vi "Read CAN Frame.vi"(8 "error in (no error)":errorcluster, 10 "Header Read":T3, 11 "BLF File In":refnum<class "Read Write BLF.lvclass">) -> (0 "error out":errorcluster, 1 "CAN Channel":u16, 2 "CAN Frame":T1 {"type" items=["CAN Data"=0, "CAN Remote"=1, "CAN Bus Error"=2, "CAN 2.0 Data"=8, "CAN FD Data"=16, "CAN FD+BRS Data"=24, "J1939 Data"=192, "Delay"=224, "Log Trigger"=225, "Start Trigger"=226]; "payload" format="%x"; "timestamp" format="%<%.7X\n%x>T"; "identifier" format="%x"}, 3 "BLF File Out":refnum<class "Read Write BLF.lvclass">)   [LabVIEW 2015, in "Read Write BLF.lvclass"]
doc: "This is the private function that will read a single <B>CAN Frame</B> given the header information of the next object position.\n\n-------------\nBrian Hoover (Hooovahh)"
uses:
  Read Write BLF.lvclass
  Controls/Cluster - mHeaderBase.ctl
  Controls/Enum - Read Object Types.ctl
  Controls/Cluster - CAN Frame.ctl
  Controls/Enum - CAN Data Type.ctl
  Read Write BLF.lvclass/Read Write BLF.ctl
  Controls/Cluster - CAN Message.ctl
  Controls/Cluster - mHeader.ctl
  <vilib>/Utility/error.llb/Error Cluster From Error Code.vi
  <vilib>/Utility/file.llb/Application Directory.vi
  <vilib>/ErrorRing/Error Ring.xnode
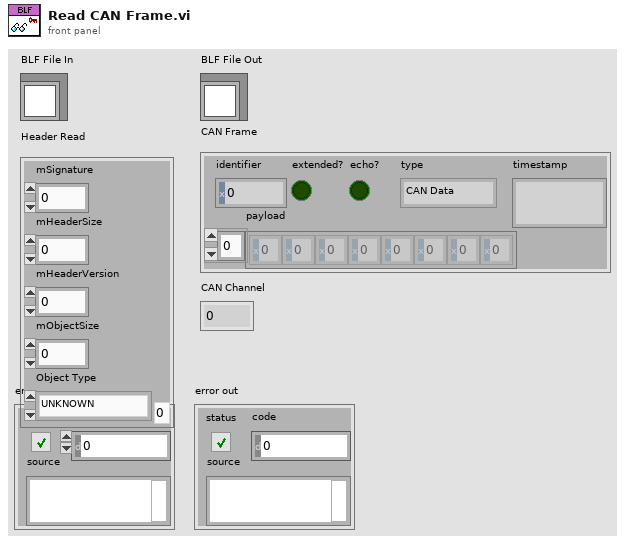
[diagram p1: front panel]
types:
  T1 = typedef "Read Write BLF.lvclass/Cluster - CAN Frame.ctl" = cluster{"timestamp":timestamp, "payload":u8[], "identifier":u32, "extended?":bool, "echo?":bool, "type":T2}
  T2 = typedef "Read Write BLF.lvclass/Enum - CAN Data Type.ctl" = u8
  T3 = typedef "Read Write BLF.lvclass/Cluster - mHeaderBase.ctl" = cluster{"mSignature":u32, "mHeaderSize":u16, "mHeaderVersion":u16, "mObjectSize":u32, "Object Type":T4}
  T4 = typedef "Read Write BLF.lvclass/Enum - Read Object Types.ctl" = enum32{"UNKNOWN", "CAN_MESSAGE", "CAN_ERROR", "CAN_OVERLOAD", "CAN_STATISTIC", "APP_TRIGGER", "ENV_INTEGER", "ENV_DOUBLE", "ENV_STRING", "ENV_DATA", "LOG_CONTAINER", "LIN_MESSAGE", "LIN_CRC_ERROR", "LIN_DLC_INFO", "LIN_RCV_ERROR", "LIN_SND_ERROR", "LIN_SLV_TIMEOUT", "LIN_SCHED_MODCH", "LIN_SYN_ERROR", "LIN_BAUDRATE", "LIN_SLEEP", "LIN_WAKEUP", "MOST_SPY", "MOST_CTRL", "MOST_LIGHTLOCK", "MOST_STATISTIC", "reserved_1", "reserved_2", "reserved_3", "FLEXRAY_DATA", "FLEXRAY_SYNC", "CAN_DRIVER_ERROR", "MOST_PKT", "MOST_PKT2", "MOST_HWMODE", "MOST_REG", "MOST_GENREG", "MOST_NETSTATE", "MOST_DATALOST", "MOST_TRIGGER", "FLEXRAY_CYCLE", "FLEXRAY_MESSAGE", "LIN_CHECKSUM_INFO", "LIN_SPIKE_EVENT", "CAN_DRIVER_SYNC", "FLEXRAY_STATUS", "GPS_EVENT", "FR_ERROR", "FR_STATUS", "FR_STARTCYCLE", "FR_RCVMESSAGE", "REALTIMECLOCK", "AVAILABLE2", "AVAILABLE3", "LIN_STATISTIC", "J1708_MESSAGE", "J1708_VIRTUAL_MSG", "LIN_MESSAGE2", "LIN_SND_ERROR2", "LIN_SYN_ERROR2", "LIN_CRC_ERROR2", "LIN_RCV_ERROR2", "LIN_WAKEUP2", "LIN_SPIKE_EVENT2", "LIN_LONG_DOM_SIG", "APP_TEXT", "FR_RCVMESSAGE_EX", "MOST_STATISTICEX", "MOST_TXLIGHT", "MOST_ALLOCTAB", "MOST_STRESS", "ETHERNET_FRAME", "SYS_VARIABLE", "CAN_ERROR_EXT", "CAN_DRIVER_ERROR_EXT", "LIN_LONG_DOM_SIG2", "MOST_150_MESSAGE", "MOST_150_PKT", "MOST_ETHERNET_PKT", "MOST_150_MESSAGE_FRAGMENT", "MOST_150_PKT_FRAGMENT", "MOST_ETHERNET_PKT_FRAGMENT", "MOST_SYSTEM_EVENT", "MOST_150_ALLOCTAB", "MOST_50_MESSAGE", "MOST_50_PKT", "CAN_MESSAGE2", "LIN_UNEXPECTED_WAKEUP", "LIN_SHORT_OR_SLOW_RESPONSE", "LIN_DISTURBANCE_EVENT", "SERIAL_EVENT", "OVERRUN_ERROR", "EVENT_COMMENT", "WLAN_FRAME", "WLAN_STATISTIC", "MOST_ECL", "GLOBAL_MARKER", "AFDX_FRAME", "AFDX_STATISTIC", "KLINE_STATUSEVENT", "CAN_FD_MESSAGE", "CAN_FD_MESSAGE_64", "ETHERNET_RX_ERROR", "ETHERNET_STATUS", "CAN_FD_ERROR_64", "LIN_SHORT_OR_SLOW_RESPONSE2", "AFDX_STATUS", "AFDX_BUS_STATISTIC"}
  T5 = typedef "Read Write BLF.lvclass/Cluster - CAN Message.ctl" = cluster{"mHeader":T6, "mChannel":u16, "mFlags":u8, "mDLC":u8, "mID":u32, "mData":cluster{"mData[0]":u8, "mData[1]":u8, "mData[2]":u8, "mData[3]":u8, "mData[4]":u8, "mData[5]":u8, "mData[6]":u8, "mData[7]":u8}}
  T6 = typedef "Read Write BLF.lvclass/Cluster - mHeader.ctl" = cluster{"mHeaderBase":T3, "mObjectFlags":u32, "mReserved":u16, "mObjectVersion":u16, "mObjectTimeStamp":u64}
  T7 = cluster{"mData[0]":u8, "mData[1]":u8, "mData[2]":u8, "mData[3]":u8, "mData[4]":u8, "mData[5]":u8, "mData[6]":u8, "mData[7]":u8}
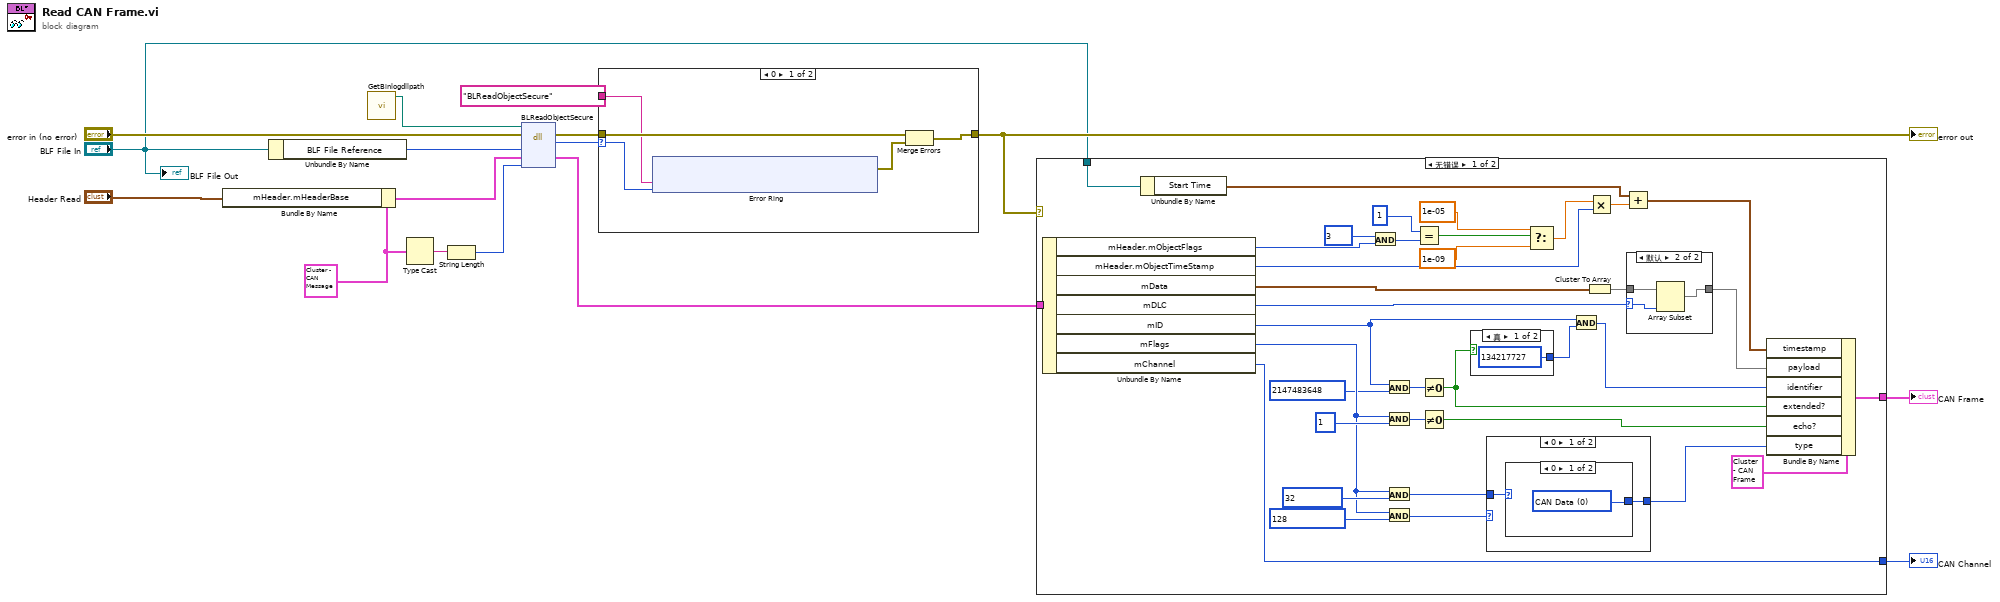
[diagram p0: block diagram]
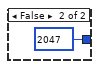
[diagram p2: hidden frame]
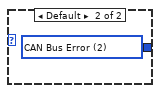
[diagram p3: hidden frame]
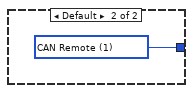
[diagram p4: hidden frame]
diagram:
  w9 = T5 {"mHeader"={"mHeaderBase"={"mSignature"=0, "mHeaderSize"=0, "mHeaderVersion"=0, "mObjectSize"=0, "Object Type"=enum."UNKNOWN"}, "mObjectFlags"=0, "mReserved"=0, "mObjectVersion"=0, "mObjectTimeStamp"=0}, "mChannel"=0, "mFlags"=0, "mDLC"=8, "mID"=0, "mData"={"mData[0]"=0, "mData[1]"=0, "mData[2]"=0, "mData[3]"=0, "mData[4]"=0, "mData[5]"=0, "mData[6]"=0, "mData[7]"=0}}
  n1 = Bundle By Name(cluster=w9, "mHeader.mHeaderBase"="Header Read") -> (w12:T5)
  n2 = Unbundle By Name("BLF File In") -> ("BLF File Reference"=w4:u32)
  n3 = call "GetBinlogdllpath.vi"() -> ("dup path"=w1:path)  [unwired: 11 in]
  n4 = Type Cast(x=w9) -> (*(type *) &x=w10:string)  [unwired: 1 in]
  n5 = String Length(string=w10) -> (length=w8:i32)
  n6 = dll-call lib="PTH2Vabs E自开发软件X-CAN项目 X-CAN离线分析平台 V2.2.8.0BLFbinlog.*" fn="BLReadObjectSecure"(path in=w1, error in="error in (no error)", "hFile"=w4, "pBase"=w12, "expectedSize"=w8) -> (error out=w14:errorcluster, "return type"=w15:i32, "pBase"=w7:T5)  [unwired: 3 in, 1 out]
  n7 = case shown="0" w15 {
    selector: w15 -> [w19 _]
    tunnel: w14 -> [w21 w30]
    tunnel: [w20 w30] -> w5
    tunnel: "BLReadObjectSecure" -> [w18 _]
    frame 0 {
      n8 = xnode "Error Ring"("参数 0"=w18, "参数 1"=w19) -> ("错误输出"=w17:errorcluster)
      n9 = Merge Errors(w21, w17) -> (w20:errorcluster)
    }
    frame Default {
    }
  }
  "error out" <- w5
  n10 = case shown="无错误" w5 {
    tunnel: w7 -> [w64 _]
    tunnel: [w43 _] -> w6
    tunnel: "BLF File In" -> [w42 _]
    tunnel: [w31 _] -> w2
    frame No Error {
      n11 = Unbundle By Name(w64) -> ("mHeader.mObjectFlags"=w40:u32, "mHeader.mObjectTimeStamp"=w46:u64, "mData"=w63:T7, "mDLC"=w61:u8, "mID"=w48:u32, "mFlags"=w54:u8, "mChannel"=w31:u16)
      n12 = Unbundle By Name(w42) -> ("Start Time"=w41:timestamp)
      n13 = And(x=u32 3, y=w40) -> (x .and. y?=w38:u32)
      n14 = And(x=w48, y=u32 2147483648) -> (x .and. y?=w50:u32)
      n15 = And(x=w54, y=u8 1) -> (x .and. y?=w58:u8)
      n16 = And(x=w54, y=u8 32) -> (x .and. y?=w52:u8)
      n17 = And(x=w54, y=u8 128) -> (x .and. y?=w53:u8)
      n18 = Equal?(x=u32 1, y=w38) -> (x = y?=w36:bool)
      n19 = Not Equal To 0?(x=w50) -> (x != 0?=w32:bool)
      n20 = Not Equal To 0?(x=w58) -> (x != 0?=w57:bool)
      n21 = case shown="真" w32 {
        tunnel: [u32 134217727 ("y") u32 2047 ("y")] -> w49
        frame True {
        }
        frame False {
        }
      }
      n22 = case shown="0" w53 {
        tunnel: [w69 w73] -> w65
        tunnel: w52 -> [w70 _]
        frame 0 {
          n23 = case shown="0" w70 {
            tunnel: [w71 w72] -> w69
            frame 0 {
              w71 = T2 0 items=["CAN Data"=0, "CAN Remote"=1, "CAN Bus Error"=2, "CAN 2.0 Data"=8, "CAN FD Data"=16, "CAN FD+BRS Data"=24, "J1939 Data"=192, "Delay"=224, "Log Trigger"=225, "Start Trigger"=226] ("type")
            }
            frame Default {
              w72 = T2 2 items=["CAN Data"=0, "CAN Remote"=1, "CAN Bus Error"=2, "CAN 2.0 Data"=8, "CAN FD Data"=16, "CAN FD+BRS Data"=24, "J1939 Data"=192, "Delay"=224, "Log Trigger"=225, "Start Trigger"=226] ("type")
            }
          }
        }
        frame Default {
          w73 = T2 1 items=["CAN Data"=0, "CAN Remote"=1, "CAN Bus Error"=2, "CAN 2.0 Data"=8, "CAN FD Data"=16, "CAN FD+BRS Data"=24, "J1939 Data"=192, "Delay"=224, "Log Trigger"=225, "Start Trigger"=226] ("type")
        }
      }
      n24 = Select(t=1e-05, s=w36, f=1e-09) -> (s? t:f=w34:dbl)
      n25 = And(x=w48, y=w49) -> (x .and. y?=w47:u32)
      n26 = Cluster To Array(cluster=w63) -> (array=w62:u8[])
      n27 = Multiply(x=w34, y=w46) -> (x*y=w45:dbl)
      n28 = Add(x=w41, y=w45) -> (x+y=w44:timestamp)
      n29 = case shown="默认" w61 {
        selector: w61 -> [_ w76]
        tunnel: w62 -> [w74 w77]
        tunnel: [w74 w75] -> w60
        frame 0 {
        }
        frame Default {
          n30 = Array Subset(array=w77, length=w76) -> (w75:u8[])  [unwired: 1 in]
        }
      }
      n31 = Bundle By Name(cluster=T1 {"timestamp"=timestamp(0 s since 1904-01-01), "payload"=[], "identifier"=0, "extended?"=FALSE, "echo?"=FALSE, "type"=0} ("CAN frame"), "timestamp"=w44, "payload"=w60, "identifier"=w47, "extended?"=w32, "echo?"=w57, "type"=w65) -> (w43:T1)
    }
    frame Error {
    }
  }
  "CAN Frame" <- w6
  "CAN Channel" <- w2
  "BLF File Out" <- "BLF File In"
